vi "openDocuement.vi"(8 "error in (no error)":errorcluster, 11 "Document in":refnum<class "Document.lvclass">) -> (0 "error out":errorcluster, 3 "Document out":refnum<class "Document.lvclass">)   [LabVIEW 2020, in "LabVIEW NPOI.lvlib" / "Document.lvclass"]
doc: "Protected dynamic dispatch method to open the <b>Document</b> file located at <b>File Path</b> for reading."
uses:
  Document.lvclass
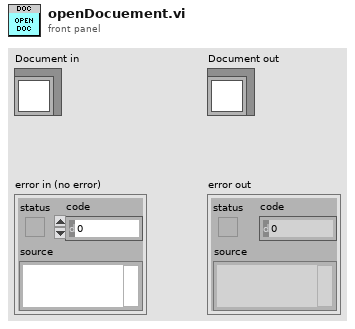
[diagram p1: front panel]
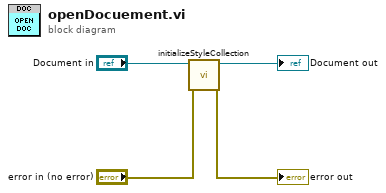
[diagram p0: block diagram]
diagram:
  n1 = call-dynamic "initializeStyleCollection.vi"("error in (no error)"="error in (no error)", "Document in"="Document in") -> ("error out"=→"error out":errorcluster, "Document out"=→"Document out":refnum<class "Document.lvclass">)  [unwired: 8 in]
